vi "ResetTime.vi"(8 "error in (no error)":errorcluster, 10 "enabled":bool, 11 "SnakeSwitch in":refnum<class "SnakeSwitch.lvclass">) -> (0 "error out":errorcluster, 3 "SnakeSwitch out":refnum<class "SnakeSwitch.lvclass">)   [LabVIEW 2019, in "RT_Game.lvlib" / "SnakeSwitch.lvclass"]
uses:
  SnakeSwitch.lvclass
  SnakeSwitch.lvclass/SnakeSwitch.ctl
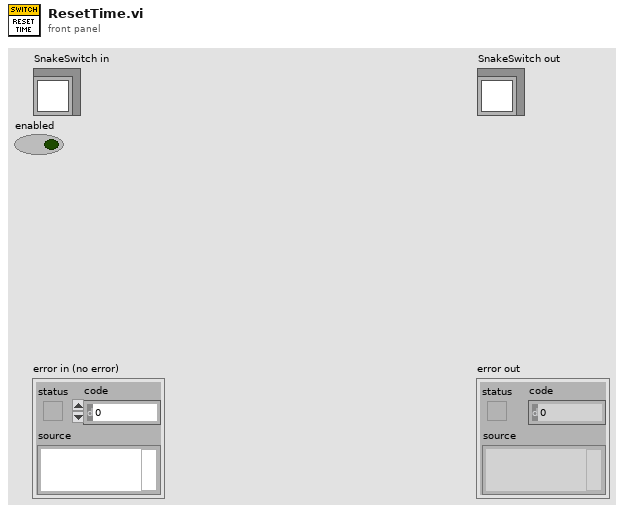
[diagram p1: front panel]
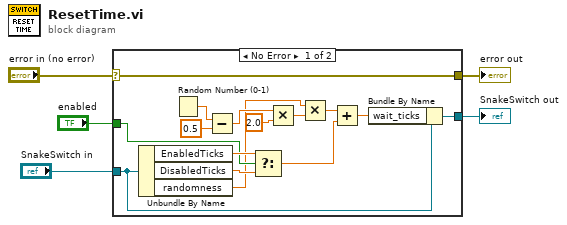
[diagram p0: block diagram]
diagram:
  n1 = case shown="No Error" "error in (no error)" {
    selector: "error in (no error)" -> [w20 w22]
    tunnel: [w20 w22] -> w4
    tunnel: [w15 w21] -> w2
    tunnel: "SnakeSwitch in" -> [w19 w21]
    tunnel: "enabled" -> [w16 _]
    frame No Error {
      n2 = Unbundle By Name(w19) -> ("EnabledTicks"=w18:dbl, "DisabledTicks"=w17:dbl, "randomness"=w7:dbl)
      n3 = Random Number (0-1)() -> (number: 0 to 1=w12:dbl)
      n4 = Subtract(x=w12, y=0.5) -> (x-y=w10:dbl)
      n5 = Select(t=w18, s=w16, f=w17) -> (s? t:f=w14:dbl)
      n6 = Multiply(x=w10, y=2.0) -> (x*y=w8:dbl)
      n7 = Multiply(x=w7, y=w8) -> (x*y=w6:dbl)
      n8 = Add(x=w6, y=w14) -> (x+y=w13:dbl)
      n9 = Bundle By Name(cluster=w19, "wait_ticks"=w13) -> (w15:refnum<class "SnakeSwitch.lvclass">)
    }
    frame Error {
    }
  }
  "error out" <- w4
  "SnakeSwitch out" <- w2
